vi "set Primary Weapon.vi"(10 "Primary Weapon":bool, 11 "Control State in":refnum<class "Control State.lvclass">) -> (3 "Control State out":refnum<class "Control State.lvclass">)   [LabVIEW 2021, in "Control State.lvclass"]
uses:
  Control State.lvclass
  Control State.lvclass/Control State.ctl
  Button State.ctl
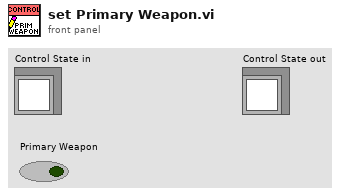
[diagram p1: front panel]
types:
  T1 = typedef "Control State.lvclass/Button State.ctl" = enum16{"Undefined", "Pressed", "Released", "Held", "Not Held"}
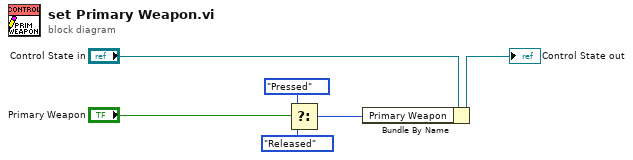
[diagram p0: block diagram]
diagram:
  n1 = Select(t=Button_State."Pressed" ("Thrust"), s="Primary Weapon", f=Button_State."Released" ("Thrust")) -> (s? t:f=w2:T1)
  n2 = Bundle By Name(cluster="Control State in", "Primary Weapon"=w2) -> (→"Control State out":refnum<class "Control State.lvclass">)
